vi "ziModGetImpedanceData.vi"(8 "Error In":errorcluster, 10 "ModResults":T3, 11 "ModHandle In":T6 {"ModHandle" format="0x%08x"; "Conn" format="0x%08x"}) -> (0 "Error Out":errorcluster, 1 "ModImpDataGrid":T1[](array[typedef]), 2 "ModImpData":T2[](array[typedef]), 3 "ModHandle Out":T6 {"ModHandle" format="0x%08x"; "Conn" format="0x%08x"})   [LabVIEW 2009, in "Zurich Instruments LabOne.lvlib"]
doc: "Use this vi to get Impedance Data from a ModResult returned from ziModGetNextNode.vi. It returns an array of Impedance Data."
uses:
  <instrlib>/Zurich Instruments LabOne/Zurich Instruments LabOne.lvlib
  <instrlib>/Zurich Instruments LabOne/Public/Modules/ziTypeModHandle.ctl
  <instrlib>/Zurich Instruments LabOne/Public/Modules/ziTypeModResults.ctl
  <instrlib>/Zurich Instruments LabOne/Public/Data/ziTypePollType.ctl
  <instrlib>/Zurich Instruments LabOne/Public/Modules/ziTypeModGenericHeader.ctl
  <instrlib>/Zurich Instruments LabOne/Public/Data/ziTypeImpedanceSample.ctl
  <instrlib>/Zurich Instruments LabOne/Public/Data/ziTypeImpedanceSampleGrid.ctl
  <instrlib>/Zurich Instruments LabOne/Public/Data/ziTypeDoubleDataTS.ctl
  <instrlib>/Zurich Instruments LabOne/Private/ziLV32.dll
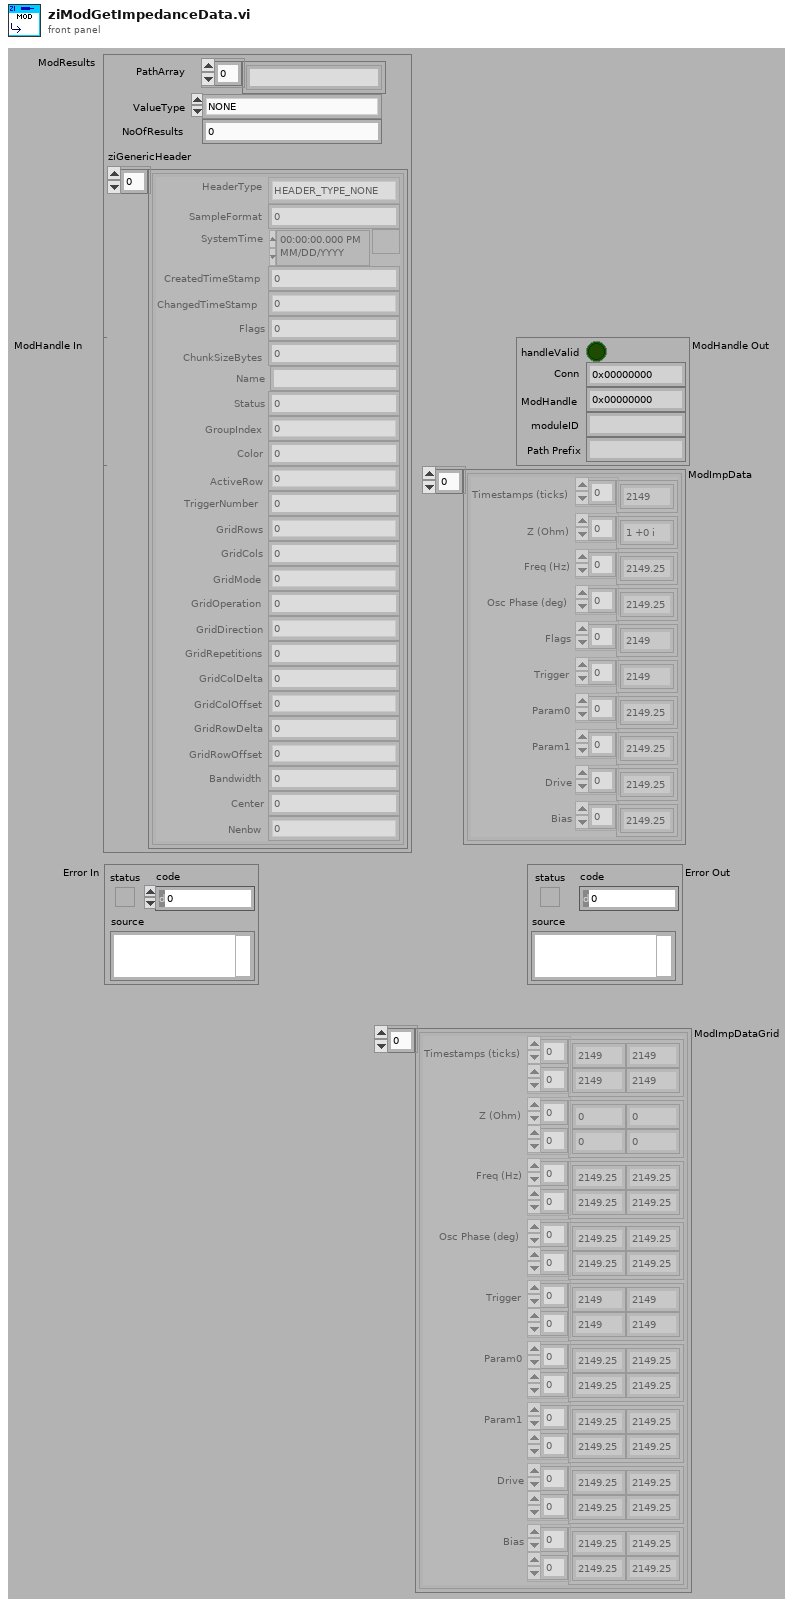
[diagram p1: front panel]
types:
  T1 = typedef "Zurich Instruments LabOne.lvlib/ziTypeImpedanceSampleGrid.ctl" = cluster{"Timestamps (ticks)":u64[][], "Z (Ohm)":cdb[][], "Freq (Hz)":dbl[][], "Osc Phase (deg)":dbl[][], "Trigger":u32[][], "Param0":dbl[][], "Param1":dbl[][], "Drive":dbl[][], "Bias":dbl[][]}
  T2 = typedef "Zurich Instruments LabOne.lvlib/ziTypeImpedanceSample.ctl" = cluster{"Timestamps (ticks)":u64[], "Z (Ohm)":cdb[], "Freq (Hz)":dbl[], "Osc Phase (deg)":dbl[], "Flags":u32[], "Trigger":u32[], "Param0":dbl[], "Param1":dbl[], "Drive":dbl[], "Bias":dbl[]}
  T3 = typedef "Zurich Instruments LabOne.lvlib/ziTypeModResults.ctl" = cluster{"PathArray":string[], "ValueType":T4, "NoOfResults":u64, "ziGenericHeader":T5[]}
  T4 = typedef "Zurich Instruments LabOne.lvlib/ziTypePollType.ctl" = enum16{"NONE", "DOUBLE_DATA", "INTEGER_DATA", "DEMOD_SAMPLE", "SCOPE_WAVE_HF2", "AUXIN_SAMPLE", "DIO_SAMPLE", "BYTE_ARRAY", "PWA_WAVE", "9", "10", "11", "12", "13", "14", "15", "TREE_CHANGE_DEPRI", "17", "ERROR", "19", "20", "21", "22", "23", "24", "25", "26", "27", "28", "29", "30", "31", "DOUBLE_DATA_TS", "INTEGER_DATA_TS", "34", "SCOPE_WAVE", "SCOPE_WAVE_EX", "37", "BYTE_ARRAY_TS", "39", "40", "41", "42", "43", "44", "45", "CNT_DATA", "47", "TREE_CHANGE", "49", "50", "51", "52", "53", "54", "55", "56", "57", "58", "59", "60", "61", "62", "63", "SWEEPER_DATA", "SPECTRUM_DATA", "ADVISOR_DATA", "VECTOR_DATA", "IMP_DATA"}
  T5 = typedef "Zurich Instruments LabOne.lvlib/ziTypeModGenericHeader.ctl" = cluster{"HeaderType":enum8{"HEADER_TYPE_NONE", "HEADER_TYPE_SWTRIGGER", "HEADER_TYPE_SWEEPER"}, "SampleFormat":u8, "SystemTime":timestamp, "CreatedTimeStamp":u64, "ChangedTimeStamp":u64, "Flags":u32, "ChunkSizeBytes":u64, "Name":string, "Status":u32, "GroupIndex":u32, "Color":u32, "ActiveRow":u32, "TriggerNumber":u64, "GridRows":u32, "GridCols":u32, "GridMode":u32, "GridOperation":u32, "GridDirection":u32, "GridRepetitions":u32, "GridColDelta":dbl, "GridColOffset":dbl, "GridRowDelta":dbl, "GridRowOffset":dbl, "Bandwidth":dbl, "Center":dbl, "Nenbw":dbl}
  T6 = typedef "Zurich Instruments LabOne.lvlib/ziTypeModHandle.ctl" = cluster{"handleValid":bool, "Conn":u64, "ModHandle":u64, "moduleID":string, "Path Prefix":string}
  T7 = typedef "Zurich Instruments LabOne.lvlib/ziTypeDoubleDataTS.ctl" = cluster{"Timestamp (ticks)":u64[], "Value":dbl[]}
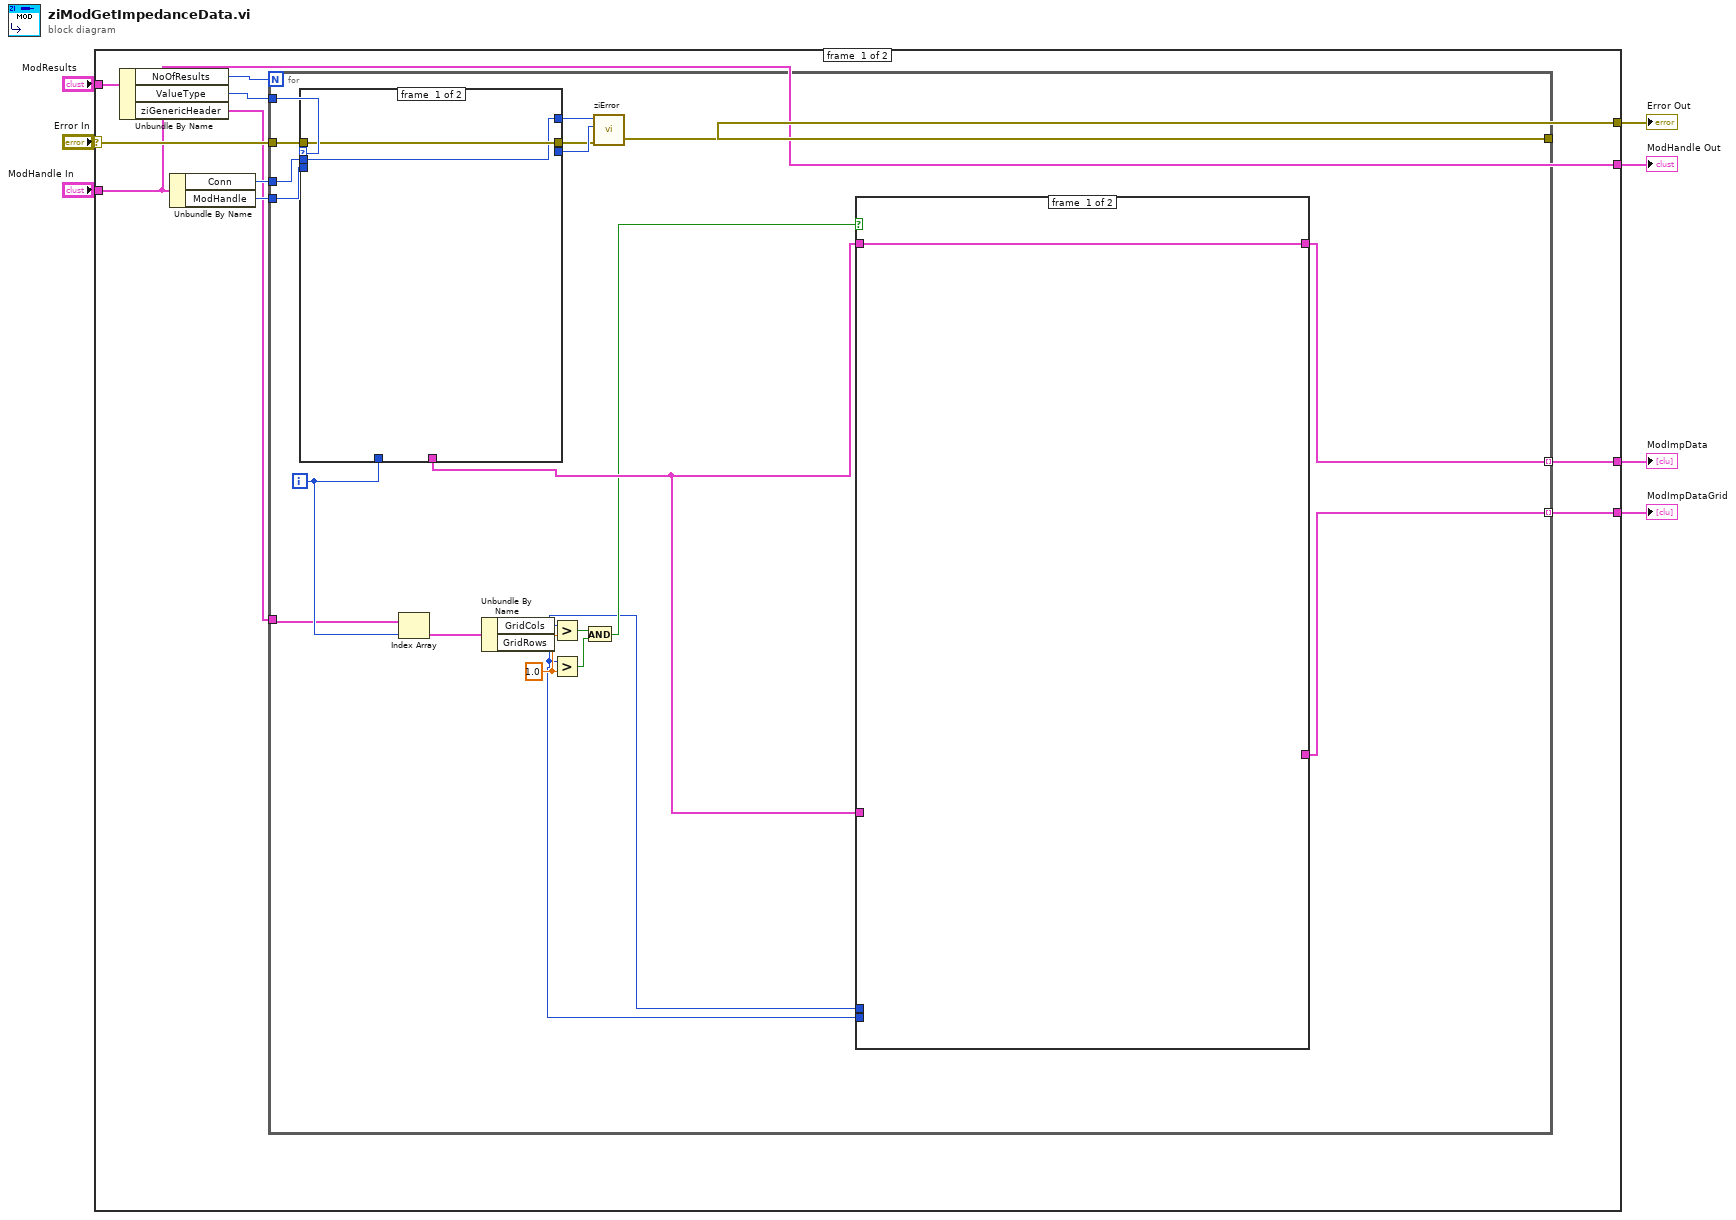
[diagram p0: block diagram]
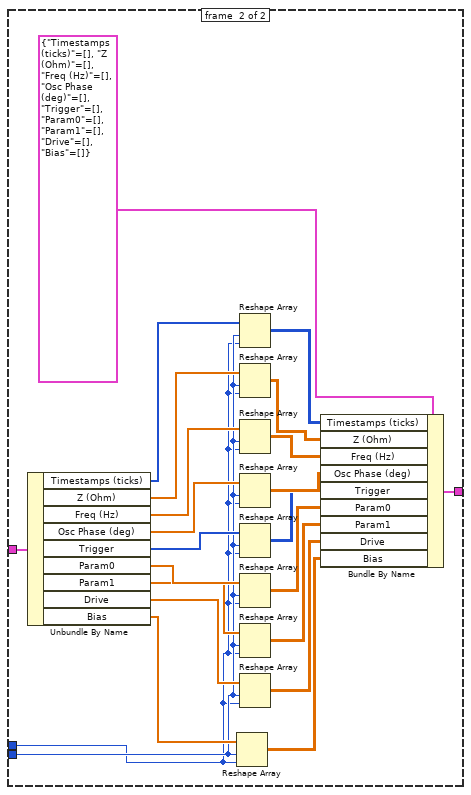
[diagram p2: hidden frame]
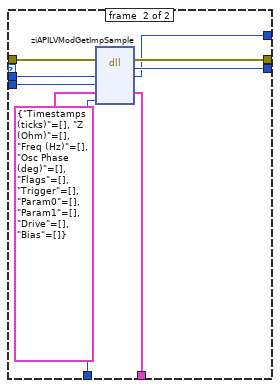
[diagram p3: hidden frame]
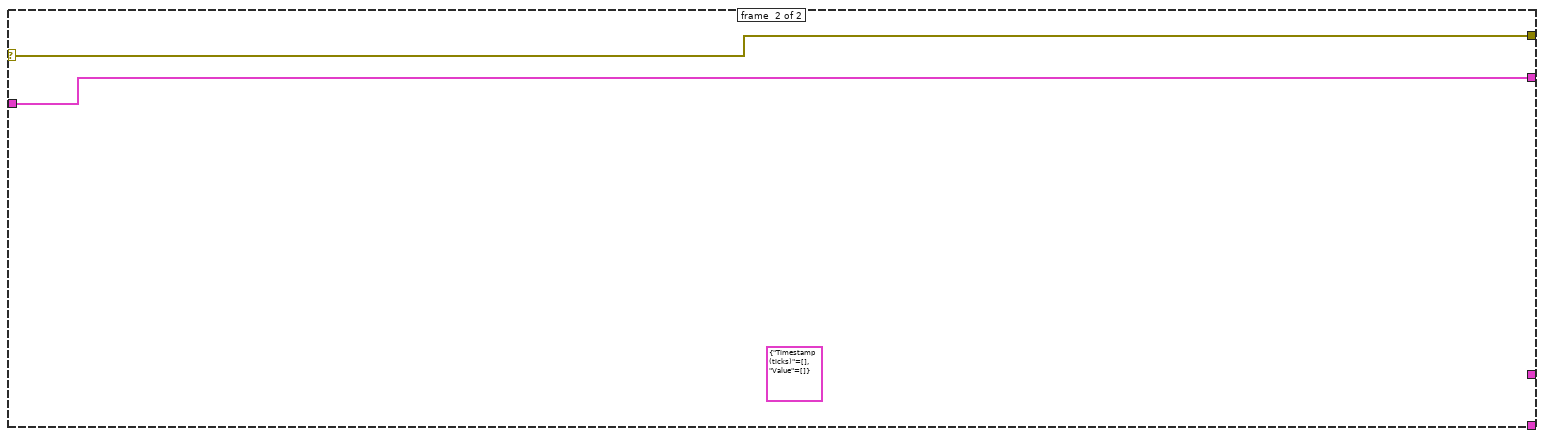
[diagram p4: hidden frame]
diagram:
  n1 = case shown="No Error" "Error In" {
    selector: "Error In" -> [w13 w74]
    tunnel: [w14 w74] -> w3
    tunnel: [w12 w75] -> w6
    tunnel: "ModHandle In" -> [w12 w75]
    tunnel: "ModResults" -> [w16 _]
    tunnel: [w10 _] -> w2
    tunnel: [w8 _] -> w1
    frame #0 {
      n2 = Unbundle By Name(w16) -> ("NoOfResults"=w15:u64, "ValueType"=w11:T4, "ziGenericHeader"=w9:T5[])
      n3 = Unbundle By Name(w12) -> ("Conn"=w18:u64, "ModHandle"=w17:u64)
      n4 = for {
        N: w15 -> [_]
        tunnel: w18 -> [w38]
        tunnel: w17 -> [w37]
        tunnel: [w36] -> w14
        tunnel: w13 -> [w33]
        tunnel: w11 -> [w32]
        tunnel: [w30] -> w10 mode=indexing
        tunnel: w9 -> [w20]
        tunnel: [w24] -> w8 mode=indexing
        i -> [w21]
        w28 = 1.0 ("y")
        n5 = case shown="\"IMP_DATA\"" w32 {
          tunnel: w38 -> [w63 w73]
          tunnel: w37 -> [_ w72]
          tunnel: w21 -> [_ w71]
          tunnel: [_ w70] -> w35
          tunnel: [w64 w69] -> w34
          tunnel: w33 -> [w64 w68]
          tunnel: [_ w67] -> w29
          tunnel: [w63 w66] -> w31
          frame #0 {
          }
          frame #1 {
            n6 = dll-call lib="C:/Program Files (x86)/National Instruments/LabVIEW 2009/instr.lib/Zurich Instruments LabOne/Private/ziLV*.*" fn="ziAPILVModGetImpSample"(error in=w68, "Conn"=w73, "ModHandle"=w72, "DEMODData"=T2 {"Timestamps (ticks)"=[], "Z (Ohm)"=[], "Freq (Hz)"=[], "Osc Phase (deg)"=[], "Flags"=[], "Trigger"=[], "Param0"=[], "Param1"=[], "Drive"=[], "Bias"=[]}, "chunk_idx"=w71) -> (error out=w69:errorcluster, "return type"=w70:u32, "Conn"=w66:u64, "DEMODData"=w67:T2)  [unwired: 4 in, 1 out]
          }
        }
        n7 = Index Array(array=w20, index=w21) -> (element=w19:T5)
        n8 = Unbundle By Name(w19) -> ("GridCols"=w22:u32, "GridRows"=w23:u32)
        n9 = Greater?(x=w22, y=w28) -> (0:w26:bool)
        n10 = Greater?(x=w23, y=w28) -> (0:w27:bool)
        n11 = And(x=w26, y=w27) -> (x .and. y?=w25:bool)
        n12 = call <instrlib>:"ziError.vi"("Conn"=w31, "ziErrorCode"=w35, "Error In"=w34) -> ("Error Out"=w36:errorcluster)  [unwired: 2 in, 1 out]
        n13 = case shown="True" w25 {
          tunnel: w29 -> [_ w62]
          tunnel: w29 -> [w39 _]
          tunnel: [w39 _] -> w30
          tunnel: [_ w53] -> w24
          tunnel: w23 -> [_ w42]
          tunnel: w22 -> [_ w41]
          frame #0 {
          }
          frame #1 {
            n14 = Unbundle By Name(w62) -> ("Timestamps (ticks)"=w61:u64[], "Z (Ohm)"=w60:cdb[], "Freq (Hz)"=w59:dbl[], "Osc Phase (deg)"=w58:dbl[], "Trigger"=w57:u32[], "Param0"=w56:dbl[], "Param1"=w55:dbl[], "Drive"=w54:dbl[], "Bias"=w43:dbl[])
            n15 = Reshape Array(w43, w42, w41) -> (w44:dbl[][])
            n16 = Reshape Array(w61, w42, w41) -> (w49:u64[][])
            n17 = Reshape Array(w60, w42, w41) -> (w40:cdb[][])
            n18 = Reshape Array(w59, w42, w41) -> (w48:dbl[][])
            n19 = Reshape Array(w58, w42, w41) -> (w47:dbl[][])
            n20 = Reshape Array(w57, w42, w41) -> (w46:u32[][])
            n21 = Reshape Array(w56, w42, w41) -> (w45:dbl[][])
            n22 = Reshape Array(w55, w42, w41) -> (w50:dbl[][])
            n23 = Reshape Array(w54, w42, w41) -> (w51:dbl[][])
            n24 = Bundle By Name(cluster=T1 {"Timestamps (ticks)"=[], "Z (Ohm)"=[], "Freq (Hz)"=[], "Osc Phase (deg)"=[], "Trigger"=[], "Param0"=[], "Param1"=[], "Drive"=[], "Bias"=[]} ("Imp Sample"), "Timestamps (ticks)"=w49, "Z (Ohm)"=w40, "Freq (Hz)"=w48, "Osc Phase (deg)"=w47, "Trigger"=w46, "Param0"=w45, "Param1"=w50, "Drive"=w51, "Bias"=w44) -> (w53:T1)
          }
        }
      }
    }
    frame #1 {
      (unwired) T7 {"Timestamp (ticks)"=[], "Value"=[]} ("DoubleSample")
    }
  }
  "Error Out" <- w3
  "ModHandle Out" <- w6
  "ModImpData" <- w2
  "ModImpDataGrid" <- w1
